vi "Global.vi"() -> ()   [LabVIEW 2020]
uses:
  <vilib>/Utility/miscctls.llb/LVRectTypeDef.ctl
panel:
  out "IORef":refnum<vi>
  in  "FrontPanelSettingQueue":refnum<queue>
  out "UserPanelCMDQueue":refnum<queue>
  in  "SubThreadRef":refnum<vi>
  in  "DynaPanelbound":T1
  in  "ThreadCMDQueue":refnum<queue>[](array[refnum])
  in  "VittualIOName":string
  in  "SystemPauseRef":refnum<vi>
  in  "SubThreadQueue":refnum<queue>
  out "CreateSubThreadMod":refnum<queue>
  in  "ProgramName":refnum<vi>
  in  "UserFrontPanel":refnum<vi>
  out "ARCOSPanel":refnum<vi>
  out "程序":refnum<vi>
  out "MainPath":path
  out "Work Path":path
  in  "ProgramSectionRingRef":refnum<vi>
  out "ExternalModule":refnum<queue>
  out "Capture Mod":refnum<queue>
  out "System Mod":refnum<queue>
  out "緊急停止":bool
  out "DAQ Mod":refnum<queue>
  out "程式結束":bool
  out "IO Mod":refnum<queue>
  out "Motor Mod":refnum<queue>
  out "總程序編輯表":refnum<vi>
  out "COMMAND執行表":T2(array[cluster])
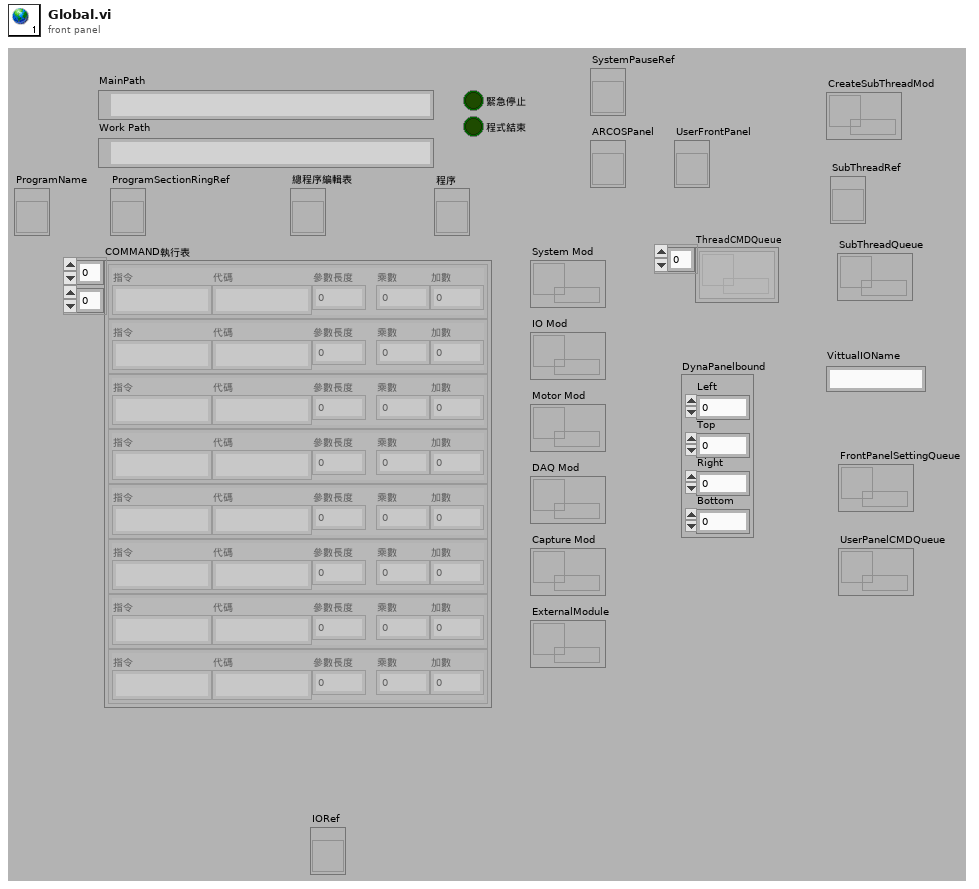
[diagram p1: front panel]
types:
  T1 = typedef "LVRectTypeDef.ctl" = cluster{"Left":i16, "Top":i16, "Right":i16, "Bottom":i16}
  T2 = cluster{"指令":string, "代碼":string, "參數長度":i32, "乘數":dbl, "加數":dbl}[][]
diagram:
